vi "CrossoverFilter.vi"() -> ()   [LabVIEW 2021]
uses:
  <vilib>/measure/matone.llb/Extract Single Tone Information 1 Chan.vi
  <resource>/objmgr/daqmx.rc
  <vilib>/measure/NI_MABase.lvlib
  <vilib>/measure/NI_MAPro.lvlib
panel:
  in  "Interval time (ms)":u32
  in  "Max freq (Hz)":dbl
  in  "Min freq (Hz)":dbl
  in  "Step (Hz)":dbl
  in  "Frequency analysis":bool
  out "Phase":cluster{"X":dbl[], "Y":dbl[]}[](graph)
  out "Amplitude":cluster{"X":dbl[], "Y":dbl[]}[](graph)
  in  "Signals graph":bool
  in  "Voltage graph":bool
  in  "Save signals":bool
  in  "Signal N samples":i32=100
  in  "Signal rate":dbl=100000.0
  out "Signals":waveform(dbl)[](graph)
  out "Simulated ao1":waveform(dbl)
  out "Simulated ao0":waveform(dbl)
  in  "Generate ao1":bool
  in  "Amplitude 1":dbl=1.0 format="%0.2p"
  in  "Amplitude 0":dbl=1.0 format="%0.2p"
  in  "Frequency 1":dbl=1000.0
  in  "Frequency 0":dbl=1000.0
  in  "Generate ao0":bool
  out "Voltage measurement":dynamicdata(graph)
  in  "Device":tag="Dev2"
  in  "Save noise":bool
  in  "Voltage N of samples":i32=100
  in  "Voltage sample rate":dbl=1000.0
  # "Channels: ai1, ai2, ai3"
  # "Channel: ai0"
  # "Function generation"
  # "Woofer"
  # "Tweeter"
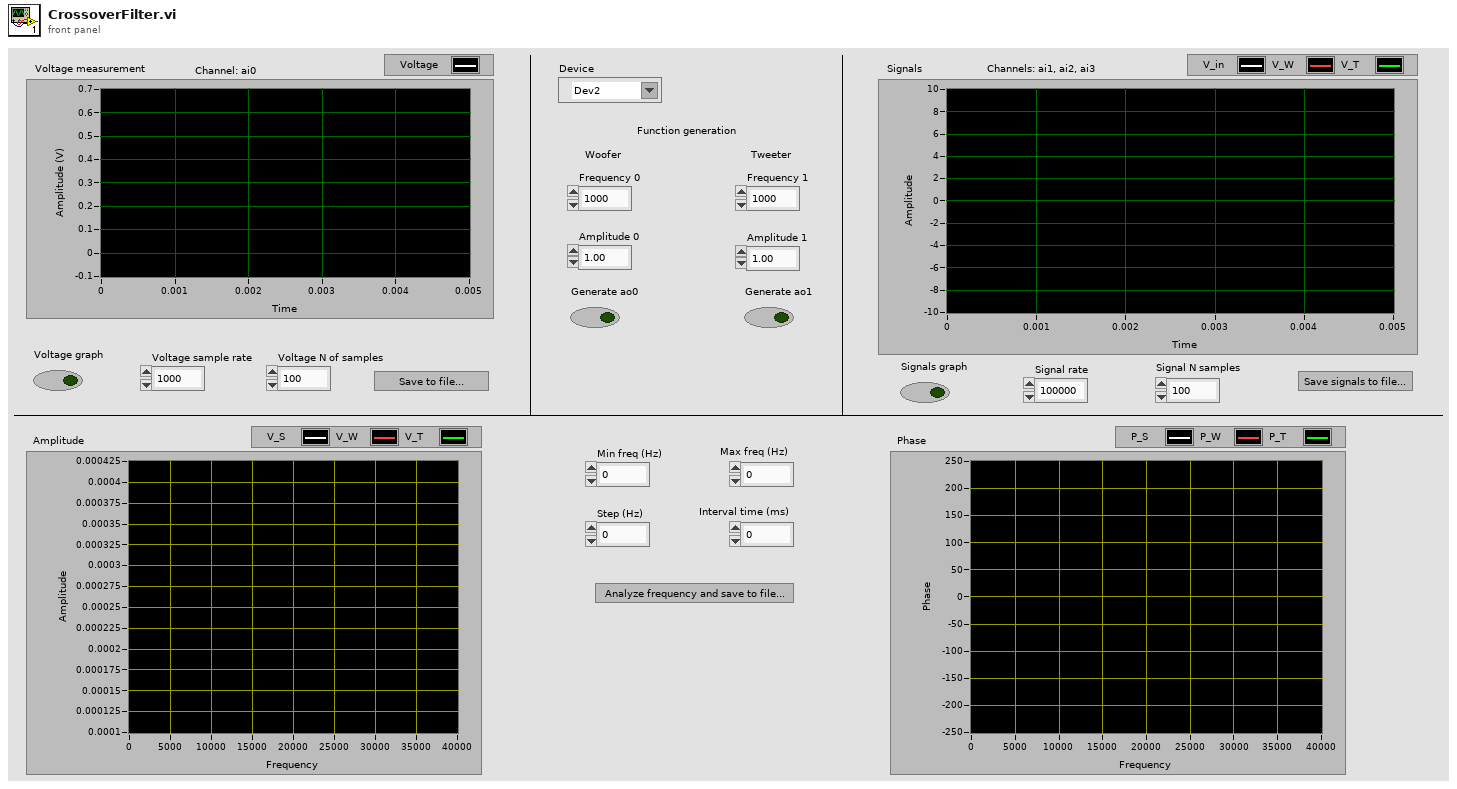
[diagram p1: front panel]
types:
  T1 = enum16{"Sine Wave", "Triangle Wave", "Square Wave", "Sawtooth Wave"}
  T2 = typedef "Semaphore RefNum" = refnum<k1>
  T3 = enum8{"Enabled", "Disabled", "Disabled and Grayed Out"}
  T4 = cluster{"detected frequency":dbl, "detected amplitude":dbl, "detected phase (deg)":dbl}
  T5 = cluster{"detected frequency":dbl, "detected amplitude":dbl, "detected phase (deg)":dbl}[][]
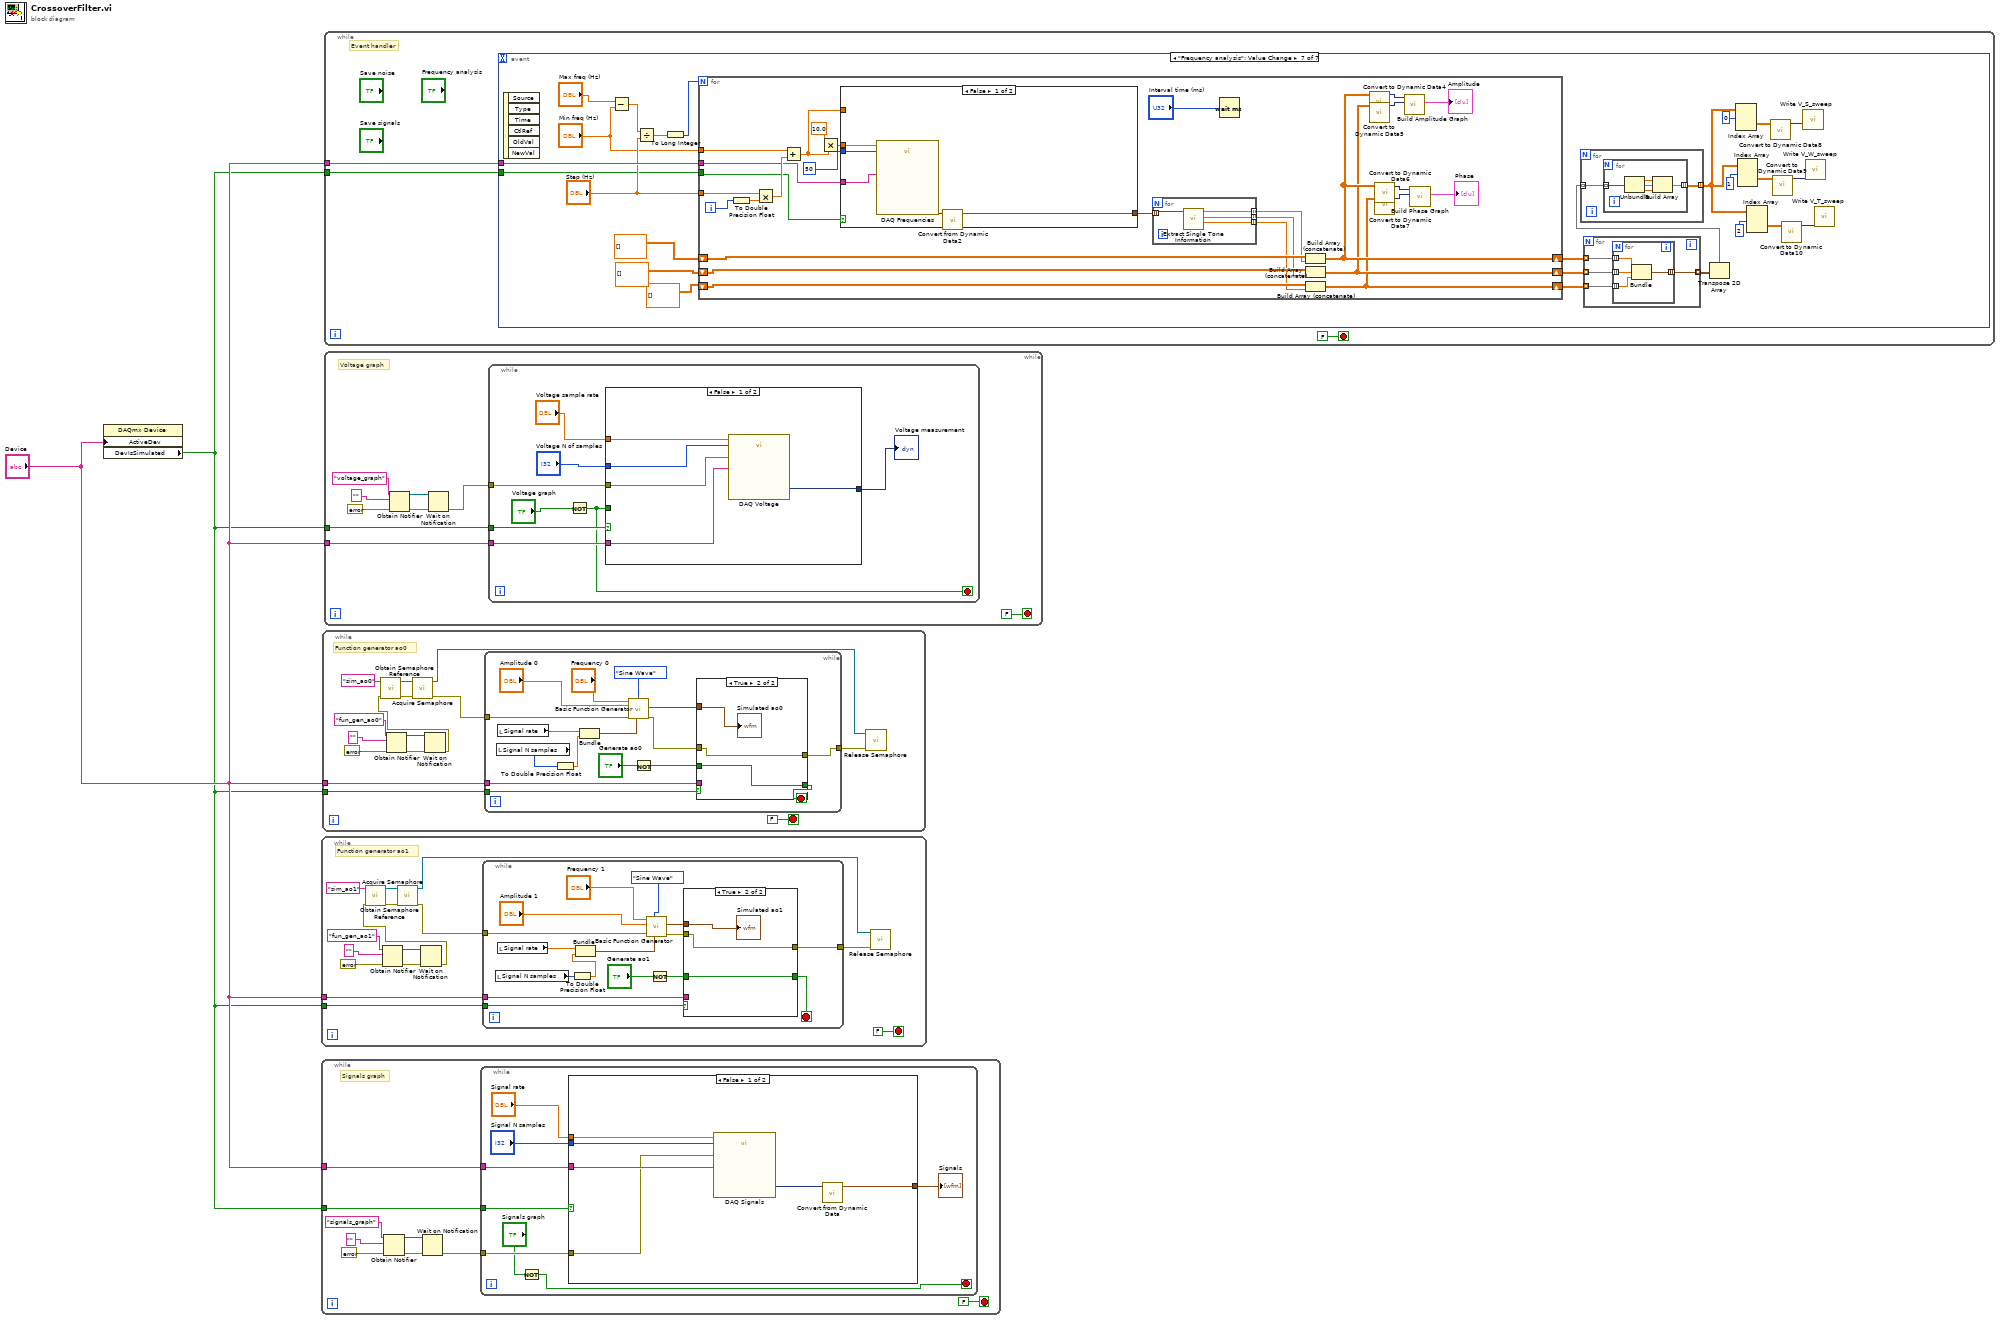
[diagram p0: block diagram]
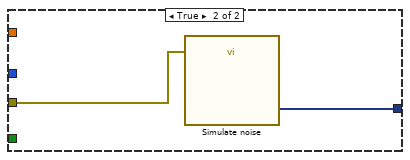
[diagram p2: hidden frame]
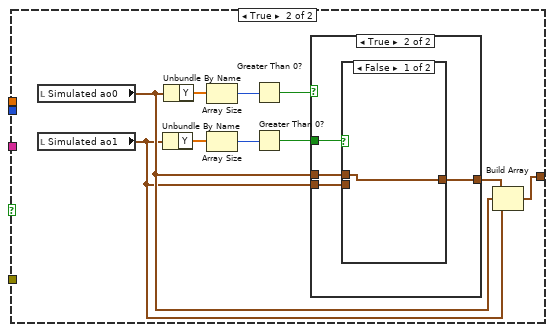
[diagram p3: hidden frame]
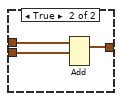
[diagram p5: hidden frame]
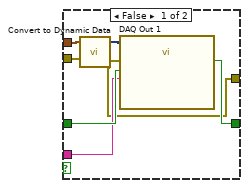
[diagram p6: hidden frame]
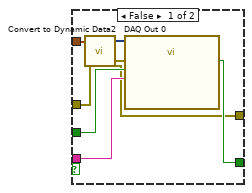
[diagram p7: hidden frame]
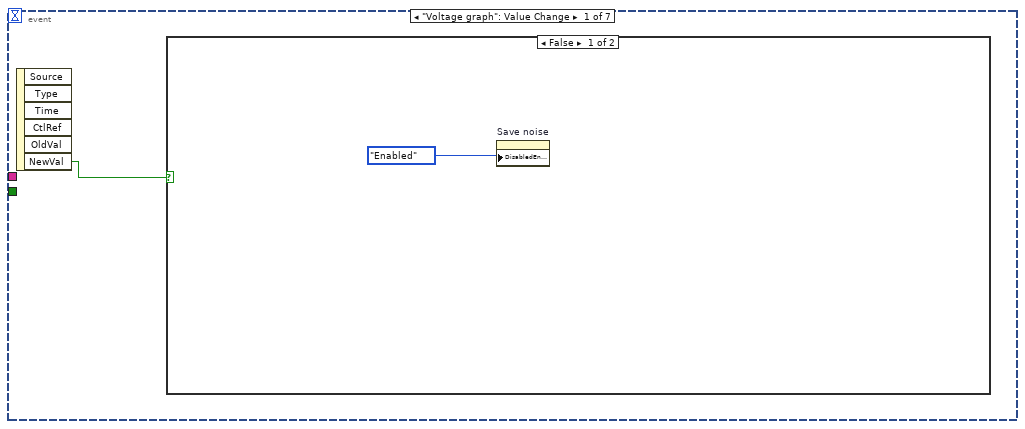
[diagram p8: hidden frame]
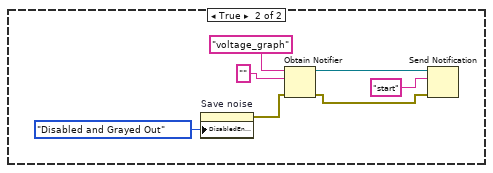
[diagram p9: hidden frame]
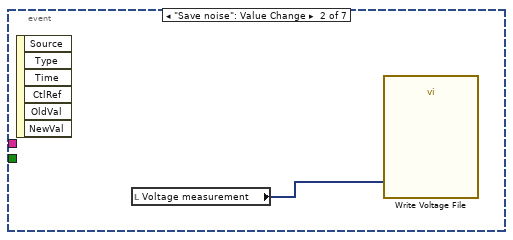
[diagram p10: hidden frame]
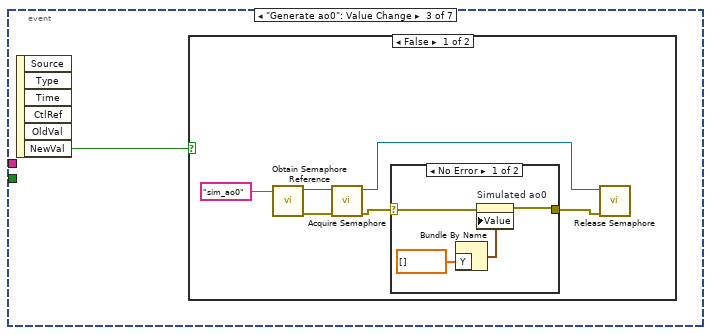
[diagram p11: hidden frame]
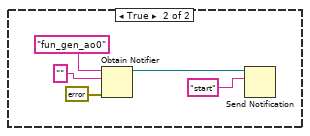
[diagram p13: hidden frame]
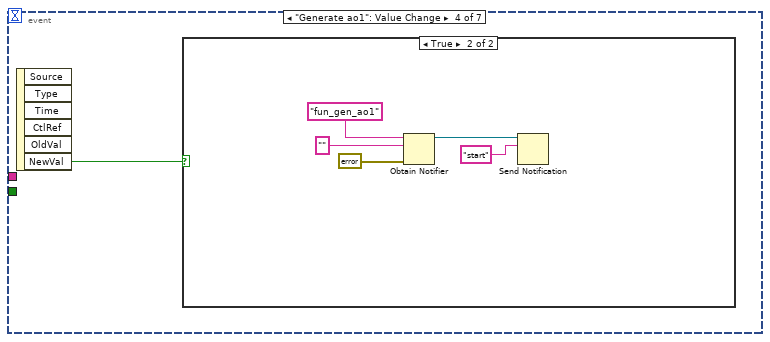
[diagram p14: hidden frame]
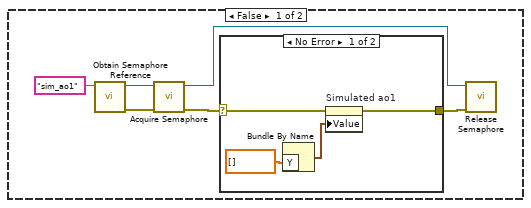
[diagram p15: hidden frame]
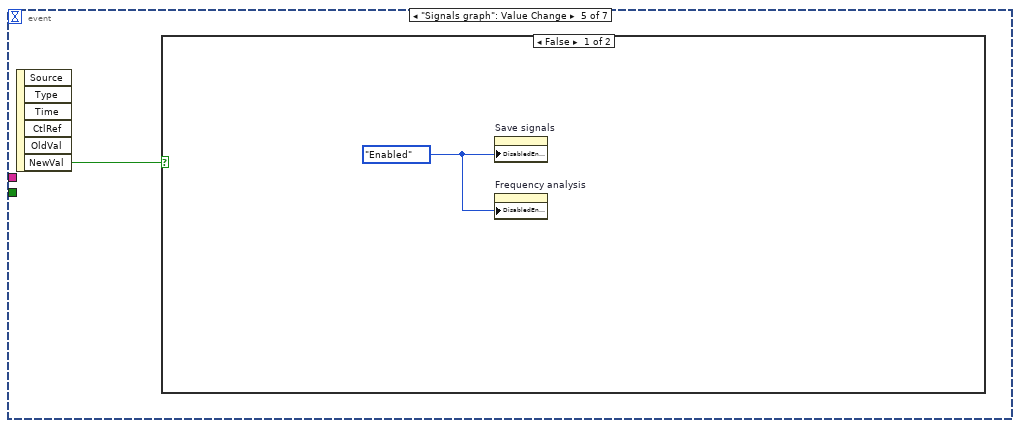
[diagram p17: hidden frame]
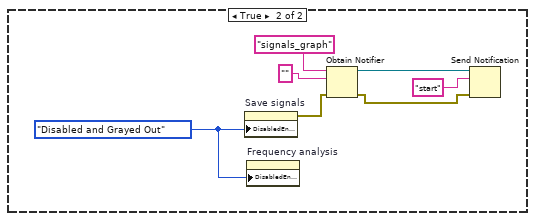
[diagram p18: hidden frame]
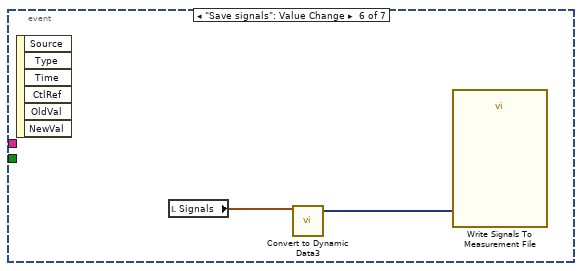
[diagram p19: hidden frame]
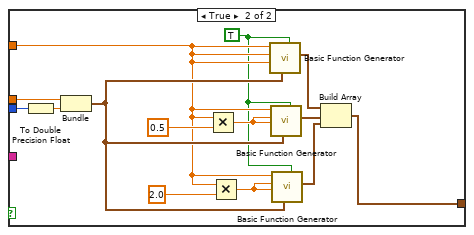
[diagram p20: hidden frame]
diagram:
  n1 = property class="DAQmx Device"("ActiveDev"="Device") -> ("DevIsSimulated"=w1:bool)  [unwired: 2 in, 2 out]
  n2 = while {
    tunnel: "Device" -> [w10]
    tunnel: w1 -> [w11]
    stop <- FALSE stop-if-true
    # "Function generator ao1"
    n3 = Obtain Notifier(name (unnamed)="fun_gen_ao1", notification data type="", error in (no error)=errorcluster {"status"=FALSE, "code"=0, "source"=""}) -> (notifier out=w16:refnum<notifier>, error out=w14:errorcluster)  [unwired: 1 in, 1 out]
    n4 = Wait on Notification(notifier=w16, error in (no error)=w14) -> (error out=w6:errorcluster)  [unwired: 2 in, 3 out]
    n5 = call <vilib>:"Obtain Semaphore Reference.vi"("error in (no error)"=w6, "name (unnamed)"="sim_ao1") -> ("error out"=w9:errorcluster, "semaphore"=w8:T2)  [unwired: 3 in, 1 out]
    n6 = call <vilib>:"Acquire Semaphore.vi"("error in (no error)"=w9, "semaphore"=w8) -> ("error out"=w5:errorcluster, "semaphore out"=w4:T2)  [unwired: 3 in, 1 out]
    n7 = while {
      tunnel: w5 -> [w30]
      tunnel: w11 -> [w28]
      tunnel: w10 -> [w27]
      tunnel: [w18] -> w3
      stop <- w32 stop-if-true
      n8 = local read "Signal N samples"() -> (w20:i32)
      n9 = local read "Signal rate"() -> (w21:dbl)
      n10 = To Double Precision Float(number=w20) -> (double precision float=w19:dbl)
      n11 = Bundle("Signal rate"=w21, w19) -> (w22:cluster{"Signal rate":dbl, dbl})  [unwired: 1 in]
      n12 = call <vilib>:"Basic Function Generator.vi"("sampling info"=w22, "signal type"=T1."Sine Wave", "error in (no error)"=w30, "amplitude"="Amplitude 1", "frequency"="Frequency 1") -> ("error out"=w24:errorcluster, "signal out"=w29:waveform(dbl))  [unwired: 4 in, 1 out]
      n13 = Not(x="Generate ao1") -> (.not. x?=w31:bool)
      n14 = case shown="True" w28 {
        tunnel: [w39 w42] -> w32
        tunnel: w31 -> [w38 w42]
        tunnel: w29 -> [w37 w41]
        tunnel: w27 -> [w35 _]
        tunnel: w24 -> [w34 w40]
        tunnel: [w34 w40] -> w18
        frame False {
          n15 = call "Convert to Dynamic Data"("Waveform"=w37) -> ("Dynamic Data Type"=w36:dynamicdata)  [unwired: 3 in]
          n16 = call "DAQ Out 1"("data"=w36, "error in"=w34, "stop (F)"=w38, "device name"=w35) -> ("stopped"=w39:bool)  [unwired: 13 in, 2 out]
        }
        frame True {
          "Simulated ao1" <- w41
        }
      }
    }
    n17 = call <vilib>:"Release Semaphore.vi"("error in (no error)"=w3, "semaphore"=w4) -> ()  [unwired: 4 in, 2 out]
  }
  n18 = while {
    tunnel: "Device" -> [w50]
    tunnel: w1 -> [w49]
    stop <- FALSE stop-if-true
    # "Signals graph"
    n19 = Obtain Notifier(name (unnamed)="signals_graph", notification data type="", error in (no error)=errorcluster {"status"=FALSE, "code"=0, "source"=""}) -> (notifier out=w48:refnum<notifier>, error out=w46:errorcluster)  [unwired: 1 in, 1 out]
    n20 = Wait on Notification(notifier=w48, error in (no error)=w46) -> (error out=w43:errorcluster)  [unwired: 2 in, 3 out]
    n21 = while {
      tunnel: w50 -> [w57]
      tunnel: w49 -> [w55]
      tunnel: w43 -> [w54]
      stop <- w52 stop-if-true
      n22 = Not(x="Signals graph") -> (.not. x?=w52:bool)
      n23 = case shown="False" w55 {
        tunnel: "Signal rate" -> [w65 _]
        tunnel: "Signal N samples" -> [w64 _]
        tunnel: w57 -> [w63 _]
        tunnel: [w61 w68] -> w56
        tunnel: w54 -> [w60 _]
        frame False {
          n24 = call "DAQ Signals"("rate"=w65, "number of samples"=w64, "error in"=w60, "device name"=w63) -> ("data"=w62:dynamicdata)  [unwired: 13 in, 2 out]
          n25 = call "Convert from Dynamic Data"("Dynamic Data Type"=w62) -> ("Array of Waveform"=w61:waveform(dbl)[])  [unwired: 3 in]
        }
        frame True {
          n26 = local read "Simulated ao0"() -> (w67:waveform(dbl))
          n27 = local read "Simulated ao1"() -> (w66:waveform(dbl))
          n28 = Unbundle By Name(w66) -> ("Y"=w74:dbl[])
          n29 = Unbundle By Name(w67) -> ("Y"=w75:dbl[])
          n30 = Array Size(array=w75) -> (size(s)=w73:i32)
          n31 = Array Size(array=w74) -> (size(s)=w72:i32)
          n32 = Greater Than 0?(x=w73) -> (x > 0?=w71:bool)
          n33 = Greater Than 0?(x=w72) -> (x > 0?=w70:bool)
          n34 = case shown="True" w71 {
            tunnel: w70 -> [_ w80]
            tunnel: w67 -> [_ w79]
            tunnel: w66 -> [w76 w78]
            tunnel: [w76 w77] -> w69
            frame False {
            }
            frame True {
              n35 = case shown="False" w80 {
                tunnel: w79 -> [w81 w84]
                tunnel: w78 -> [_ w83]
                tunnel: [w81 w82] -> w77
                frame False {
                }
                frame True {
                  n36 = Add(1:w83, 2:w84) -> (0:w82:waveform(dbl))  [unwired: 1 in, 1 out]
                }
              }
            }
          }
          n37 = Build Array(w69, w67, w66) -> (w68:waveform(dbl)[])
        }
      }
      "Signals" <- w56
    }
  }
  n38 = while {
    tunnel: "Device" -> [w92]
    tunnel: w1 -> [w93]
    stop <- FALSE stop-if-true
    # "Function generator ao0"
    n39 = Obtain Notifier(name (unnamed)="fun_gen_ao0", notification data type="", error in (no error)=errorcluster {"status"=FALSE, "code"=0, "source"=""}) -> (notifier out=w98:refnum<notifier>, error out=w96:errorcluster)  [unwired: 1 in, 1 out]
    n40 = Wait on Notification(notifier=w98, error in (no error)=w96) -> (error out=w87:errorcluster)  [unwired: 2 in, 3 out]
    n41 = call <vilib>:"Obtain Semaphore Reference.vi"("error in (no error)"=w87, "name (unnamed)"="sim_ao0") -> ("error out"=w91:errorcluster, "semaphore"=w90:T2)  [unwired: 3 in, 1 out]
    n42 = call <vilib>:"Acquire Semaphore.vi"("error in (no error)"=w91, "semaphore"=w90) -> ("error out"=w88:errorcluster, "semaphore out"=w86:T2)  [unwired: 3 in, 1 out]
    n43 = while {
      tunnel: w88 -> [w114]
      tunnel: w93 -> [w110]
      tunnel: w92 -> [w109]
      tunnel: [w100] -> w85
      stop <- w112 stop-if-true
      n44 = local read "Signal N samples"() -> (w102:i32)
      n45 = local read "Signal rate"() -> (w104:dbl)
      n46 = To Double Precision Float(number=w102) -> (double precision float=w101:dbl)
      n47 = Bundle("Signal rate"=w104, w101) -> (w103:cluster{"Signal rate":dbl, dbl})  [unwired: 1 in]
      n48 = call <vilib>:"Basic Function Generator.vi"("sampling info"=w103, "signal type"=T1."Sine Wave", "error in (no error)"=w114, "amplitude"="Amplitude 0", "frequency"="Frequency 0") -> ("error out"=w105:errorcluster, "signal out"=w113:waveform(dbl))  [unwired: 4 in, 1 out]
      n49 = Not(x="Generate ao0") -> (.not. x?=w111:bool)
      n50 = case shown="True" w110 {
        tunnel: w113 -> [w119 w123]
        tunnel: [w121 w124] -> w112
        tunnel: w111 -> [w120 w124]
        tunnel: w109 -> [w117 _]
        tunnel: w105 -> [w116 w122]
        tunnel: [w116 w122] -> w100
        frame False {
          n51 = call "Convert to Dynamic Data2"("Waveform"=w119) -> ("Dynamic Data Type"=w118:dynamicdata)  [unwired: 3 in]
          n52 = call "DAQ Out 0"("data"=w118, "error in"=w116, "stop (F)"=w120, "device name"=w117) -> ("stopped"=w121:bool)  [unwired: 13 in, 2 out]
        }
        frame True {
          "Simulated ao0" <- w123
        }
      }
    }
    n53 = call <vilib>:"Release Semaphore.vi"("error in (no error)"=w85, "semaphore"=w86) -> ()  [unwired: 4 in, 2 out]
  }
  n54 = while {
    tunnel: "Device" -> [w126]
    tunnel: w1 -> [w125]
    stop <- FALSE stop-if-true
    # "Event handler"
    n55 = event shown="[6] \"Frequency analysis\": Value Change" {
      selector: _ -> [_ _ _ _ _ _ _]
      dyn-events: _ -> [_ _ _ _ _ _ _]
      timeout: _ -> [_ _ _ _ _ _ _]
      tunnel: w126 -> [_ _ _ _ _ _ w208]
      tunnel: w125 -> [_ _ _ _ _ _ w202]
      event "Voltage graph": Value Change {
        n56 = event-data() -> ("NewVal"=w128:bool)  [unwired: 1 in, 5 out]
        n57 = case shown="False" w128 {
          frame False {
            n58 = property on="Save noise" class="Bool"("DisabledEnum"=T3."Enabled" ("Disabled")) -> ()  [unwired: 2 in, 2 out]
          }
          frame True {
            n59 = property on="Save noise" class="Bool"("DisabledEnum"=T3."Disabled and Grayed Out" ("Disabled")) -> (error out=w132:errorcluster)  [unwired: 2 in, 1 out]
            n60 = Obtain Notifier(name (unnamed)="voltage_graph", notification data type="", error in (no error)=w132) -> (notifier out=w135:refnum<notifier>, error out=w131:errorcluster)  [unwired: 1 in, 1 out]
            n61 = Send Notification(notification="start", notifier=w135, error in (no error)=w131) -> ()  [unwired: 2 out]
          }
        }
      }
      event "Save noise": Value Change {
        n62 = event-data() -> ()  [unwired: 1 in, 6 out]
        n63 = local read "Voltage measurement"() -> (w137:dynamicdata)
        n64 = call "Write Voltage File"("Signals"=w137) -> ()  [unwired: 16 in, 3 out]
      }
      event "Generate ao0": Value Change {
        n65 = event-data() -> ("NewVal"=w138:bool)  [unwired: 1 in, 5 out]
        n66 = case shown="False" w138 {
          frame False {
            n67 = call <vilib>:"Obtain Semaphore Reference.vi"("name (unnamed)"="sim_ao0") -> ("error out"=w143:errorcluster, "semaphore"=w142:T2)  [unwired: 4 in, 1 out]
            n68 = call <vilib>:"Acquire Semaphore.vi"("error in (no error)"=w143, "semaphore"=w142) -> ("error out"=w141:errorcluster, "semaphore out"=w139:T2)  [unwired: 3 in, 1 out]
            n69 = case shown="No Error" w141 {
              selector: w141 -> [w148 w149]
              tunnel: [w147 w149] -> w140
              frame No Error {
                n70 = Bundle By Name("Y"=dbl[] []) -> (w146:waveform(dbl))  [unwired: 1 in]
                n71 = property on="Simulated ao0" class="WFD (strict)"(error in=w148, "Value"=w146) -> (error out=w147:errorcluster)  [unwired: 1 in, 1 out]
              }
              frame Error {
              }
            }
            n72 = call <vilib>:"Release Semaphore.vi"("error in (no error)"=w140, "semaphore"=w139) -> ()  [unwired: 4 in, 2 out]
          }
          frame True {
            n73 = Obtain Notifier(name (unnamed)="fun_gen_ao0", notification data type="", error in (no error)=errorcluster {"status"=FALSE, "code"=0, "source"=""}) -> (notifier out=w152:refnum<notifier>)  [unwired: 1 in, 2 out]
            n74 = Send Notification(notification="start", notifier=w152) -> ()  [unwired: 1 in, 2 out]
          }
        }
      }
      event "Generate ao1": Value Change {
        n75 = event-data() -> ("NewVal"=w155:bool)  [unwired: 1 in, 5 out]
        n76 = case shown="True" w155 {
          frame False {
            n77 = call <vilib>:"Obtain Semaphore Reference.vi"("name (unnamed)"="sim_ao1") -> ("error out"=w160:errorcluster, "semaphore"=w159:T2)  [unwired: 4 in, 1 out]
            n78 = call <vilib>:"Acquire Semaphore.vi"("error in (no error)"=w160, "semaphore"=w159) -> ("error out"=w158:errorcluster, "semaphore out"=w157:T2)  [unwired: 3 in, 1 out]
            n79 = case shown="No Error" w158 {
              selector: w158 -> [w165 w166]
              tunnel: [w164 w166] -> w156
              frame No Error {
                n80 = Bundle By Name("Y"=dbl[] []) -> (w163:waveform(dbl))  [unwired: 1 in]
                n81 = property on="Simulated ao1" class="WFD (strict)"(error in=w165, "Value"=w163) -> (error out=w164:errorcluster)  [unwired: 1 in, 1 out]
              }
              frame Error {
              }
            }
            n82 = call <vilib>:"Release Semaphore.vi"("error in (no error)"=w156, "semaphore"=w157) -> ()  [unwired: 4 in, 2 out]
          }
          frame True {
            n83 = Obtain Notifier(name (unnamed)="fun_gen_ao1", notification data type="", error in (no error)=errorcluster {"status"=FALSE, "code"=0, "source"=""}) -> (notifier out=w169:refnum<notifier>)  [unwired: 1 in, 2 out]
            n84 = Send Notification(notification="start", notifier=w169) -> ()  [unwired: 1 in, 2 out]
          }
        }
      }
      event "Signals graph": Value Change {
        n85 = event-data() -> ("NewVal"=w172:bool)  [unwired: 1 in, 5 out]
        n86 = case shown="False" w172 {
          frame False {
            w173 = T3."Enabled" ("Disabled")
            n87 = property on="Save signals" class="Bool"("DisabledEnum"=w173) -> ()  [unwired: 2 in, 2 out]
            n88 = property on="Frequency analysis" class="Bool"("DisabledEnum"=w173) -> ()  [unwired: 2 in, 2 out]
          }
          frame True {
            w174 = T3."Disabled and Grayed Out" ("Disabled")
            n89 = property on="Save signals" class="Bool"("DisabledEnum"=w174) -> (error out=w175:errorcluster)  [unwired: 2 in, 1 out]
            n90 = property on="Frequency analysis" class="Bool"("DisabledEnum"=w174) -> ()  [unwired: 2 in, 2 out]
            n91 = Obtain Notifier(name (unnamed)="signals_graph", notification data type="", error in (no error)=w175) -> (notifier out=w179:refnum<notifier>, error out=w176:errorcluster)  [unwired: 1 in, 1 out]
            n92 = Send Notification(notification="start", notifier=w179, error in (no error)=w176) -> ()  [unwired: 2 out]
          }
        }
      }
      event "Save signals": Value Change {
        n93 = event-data() -> ()  [unwired: 1 in, 6 out]
        n94 = local read "Signals"() -> (w182:waveform(dbl)[])
        n95 = call "Convert to Dynamic Data3"("Array of Waveforms"=w182) -> ("Dynamic Data Type"=w181:dynamicdata)  [unwired: 3 in]
        n96 = call "Write Signals To Measurement File"("Signals"=w181) -> ()  [unwired: 16 in, 3 out]
      }
      event "Frequency analysis": Value Change {
        n97 = event-data() -> ()  [unwired: 1 in, 6 out]
        n98 = Subtract(x="Max freq (Hz)", y="Min freq (Hz)") -> (x-y=w207:dbl)
        n99 = Divide(x=w207, y="Step (Hz)") -> (x/y=w206:dbl)
        n100 = To Long Integer(number=w206) -> (32bit integer=w205:i32)
        n101 = for {
          N: w205 -> [_]
          tunnel: w208 -> [w245]
          tunnel: "Min freq (Hz)" -> [w247]
          tunnel: "Step (Hz)" -> [w250]
          tunnel: w202 -> [w240]
          shift-right: [w226] -> w197
          shift-left: dbl[][] [] -> [w232]
          shift-right: [w225] -> w196
          shift-left: dbl[][] [] -> [w230]
          shift-right: [w224] -> w195
          shift-left: dbl[][] [] -> [w228]
          i -> [w249]
          n102 = To Double Precision Float(number=w249) -> (double precision float=w248:dbl)
          n103 = Multiply(x=w250, y=w248) -> (x*y=w246:dbl)
          n104 = Add(x=w247, y=w246) -> (x+y=w239:dbl)
          n105 = Multiply(x=10.0, y=w239) -> (x*y=w244:dbl)
          n106 = case shown="False" w240 {
            tunnel: w245 -> [w256 _]
            tunnel: w244 -> [w255 w266]
            tunnel: 50 ("number of samples") -> [w254 w263]
            tunnel: [w252 w267] -> w241
            tunnel: w239 -> [_ w260]
            frame False {
              n107 = call "DAQ Frequencies"("rate"=w255, "number of samples"=w254, "device name"=w256) -> ("data"=w253:dynamicdata)  [unwired: 14 in, 2 out]
              n108 = call "Convert from Dynamic Data2"("Dynamic Data Type"=w253) -> ("Array of Waveform"=w252:waveform(dbl)[])  [unwired: 3 in]
            }
            frame True {
              w257 = TRUE ("reset signal")
              n109 = To Double Precision Float(number=w263) -> (double precision float=w264:dbl)
              n110 = Bundle(w266, w264) -> (w265:cluster{dbl, dbl})  [unwired: 1 in]
              n111 = Multiply(x=w260, y=0.5) -> (x*y=w262:dbl)
              n112 = Multiply(x=w260, y=2.0) -> (x*y=w258:dbl)
              n113 = call <vilib>:"Basic Function Generator.vi"("reset signal"=w257, "sampling info"=w265, "phase"=w260, "amplitude"=w260, "frequency"=w260) -> ("signal out"=w270:waveform(dbl))  [unwired: 4 in, 2 out]
              n114 = call <vilib>:"Basic Function Generator.vi"("reset signal"=w257, "sampling info"=w265, "phase"=w262, "amplitude"=w262, "frequency"=w260) -> ("signal out"=w269:waveform(dbl))  [unwired: 4 in, 2 out]
              n115 = call <vilib>:"Basic Function Generator.vi"("reset signal"=w257, "sampling info"=w265, "phase"=w258, "amplitude"=w258, "frequency"=w260) -> ("signal out"=w268:waveform(dbl))  [unwired: 4 in, 2 out]
              n116 = Build Array(w270, w269, w268) -> (w267:waveform(dbl)[])
            }
          }
          n117 = for {
            tunnel: w241 -> [w274] mode=indexing
            tunnel: [w273] -> w231 mode=indexing
            tunnel: [w272] -> w229 mode=indexing
            tunnel: [w271] -> w227 mode=indexing
            n118 = call-poly <vilib>:"Extract Single Tone Information.vi"("time signal in"=w274) -> ("detected phase (deg)"=w271:dbl, "detected amplitude"=w272:dbl, "detected frequency"=w273:dbl)  [unwired: 5 in, 3 out]
          }
          n119 = Wait (ms)(milliseconds to wait="Interval time (ms)") -> ()  [unwired: 1 out]
          n120 = Build Array (concatenate)(w232, w231) -> (w226:dbl[][])
          n121 = Build Array (concatenate)(w230, w229) -> (w225:dbl[][])
          n122 = Build Array (concatenate)(w228, w227) -> (w224:dbl[][])
          n123 = call "Convert to Dynamic Data4"("2D Array"=w226) -> ("Dynamic Data Type"=w235:dynamicdata)  [unwired: 3 in]
          n124 = call "Convert to Dynamic Data5"("2D Array"=w225) -> ("Dynamic Data Type"=w236:dynamicdata)  [unwired: 3 in]
          n125 = call "Convert to Dynamic Data6"("2D Array"=w226) -> ("Dynamic Data Type"=w237:dynamicdata)  [unwired: 3 in]
          n126 = call "Convert to Dynamic Data7"("2D Array"=w224) -> ("Dynamic Data Type"=w238:dynamicdata)  [unwired: 3 in]
          n127 = call "Build Amplitude Graph"("Y Input"=w236, "X Input"=w235) -> ("XY Graph"=→"Amplitude":cluster{"X":dbl[], "Y":dbl[]}[])  [unwired: 8 in, 1 out]
          n128 = call "Build Phase Graph"("Y Input"=w238, "X Input"=w237) -> ("XY Graph"=→"Phase":cluster{"X":dbl[], "Y":dbl[]}[])  [unwired: 8 in, 1 out]
        }
        n129 = for {
          tunnel: w197 -> [w219] mode=indexing
          tunnel: w196 -> [w218] mode=indexing
          tunnel: w195 -> [w217] mode=indexing
          tunnel: [w216] -> w194 mode=indexing
          n130 = for {
            tunnel: w219 -> [w223] mode=indexing
            tunnel: w218 -> [w222] mode=indexing
            tunnel: w217 -> [w221] mode=indexing
            tunnel: [w220] -> w216 mode=indexing
            n131 = Bundle("detected frequency"=w223, "detected amplitude"=w222, "detected phase (deg)"=w221) -> (w220:T4)  [unwired: 1 in]
          }
        }
        n132 = Transpose 2D Array(2D array=w194) -> (transposed array=w193:T5)
        n133 = for {
          tunnel: w193 -> [w210] mode=indexing
          tunnel: [w209] -> w183 mode=indexing
          n134 = for {
            tunnel: w210 -> [w215] mode=indexing
            tunnel: [w211] -> w209 mode=indexing
            n135 = Unbundle(w215) -> ("detected frequency"=w214:dbl, "detected amplitude"=w213:dbl, "detected phase (deg)"=w212:dbl)
            n136 = Build Array(w214, w213, w212) -> (w211:dbl[])
          }
        }
        n137 = Index Array(array=w183, index (dim 0)=0 ("index (page)")) -> (element=w191:dbl[][])  [unwired: 2 in]
        n138 = Index Array(array=w183, index (dim 0)=1 ("index (page)")) -> (element=w187:dbl[][])  [unwired: 2 in]
        n139 = Index Array(array=w183, index (dim 0)=2 ("index (page)")) -> (element=w184:dbl[][])  [unwired: 2 in]
        n140 = call "Convert to Dynamic Data8"("2D Array"=w191) -> ("Dynamic Data Type"=w190:dynamicdata)  [unwired: 3 in]
        n141 = call "Convert to Dynamic Data9"("2D Array"=w187) -> ("Dynamic Data Type"=w188:dynamicdata)  [unwired: 3 in]
        n142 = call "Convert to Dynamic Data10"("2D Array"=w184) -> ("Dynamic Data Type"=w185:dynamicdata)  [unwired: 3 in]
        n143 = call "Write V_S_sweep"("Signals"=w190) -> ()  [unwired: 16 in, 3 out]
        n144 = call "Write V_W_sweep"("Signals"=w188) -> ()  [unwired: 16 in, 3 out]
        n145 = call "Write V_T_sweep"("Signals"=w185) -> ()  [unwired: 16 in, 3 out]
      }
    }
  }
  n146 = while {
    tunnel: w1 -> [w283]
    tunnel: "Device" -> [w282]
    stop <- FALSE stop-if-true
    # "Voltage graph"
    n147 = Obtain Notifier(name (unnamed)="voltage_graph", notification data type="", error in (no error)=errorcluster {"status"=FALSE, "code"=0, "source"=""}) -> (notifier out=w280:refnum<notifier>, error out=w278:errorcluster)  [unwired: 1 in, 1 out]
    n148 = Wait on Notification(notifier=w280, error in (no error)=w278) -> (error out=w275:errorcluster)  [unwired: 2 in, 3 out]
    n149 = while {
      tunnel: w283 -> [w289]
      tunnel: w282 -> [w288]
      tunnel: w275 -> [w285]
      stop <- w286 stop-if-true
      n150 = Not(x="Voltage graph") -> (.not. x?=w286:bool)
      n151 = case shown="False" w289 {
        tunnel: [w296 w298] -> w287
        tunnel: "Voltage sample rate" -> [w295 _]
        tunnel: "Voltage N of samples" -> [w294 _]
        tunnel: w288 -> [w293 _]
        tunnel: w286 -> [_ _]
        tunnel: w285 -> [w292 w297]
        frame False {
          n152 = call "DAQ Voltage"("rate"=w295, "number of samples"=w294, "error in"=w292, "device name"=w293) -> ("data"=w296:dynamicdata)  [unwired: 13 in, 2 out]
        }
        frame True {
          n153 = call "Simulate noise"("error in (no error)"=w297) -> ("DC with Gaussian Noise"=w298:dynamicdata)  [unwired: 13 in, 1 out]
        }
      }
      "Voltage measurement" <- w287
    }
  }
